vi "LSMcontroller_v64_updatedwaveformhandling.vi"() -> ()   [LabVIEW 2015] (continued)
                        n4774 = call "correctwaveformsizetemp.vi"("new sampling frequency (Hz)"=w1792, "start"=FALSE, "reference waveforms to"=w1800, "Analog waveforms in"=w1807, "stop"=FALSE, "Digital waveforms in"=w1799) -> ("analog wf out"=w1803:waveform(dbl)[], "Digital wf out"=w1801:digitalwaveform[], "measpoints"=w1794:i32)
                        n4775 = local write "Analog Lines Plot"(w1803) -> ()
                        n4776 = call "GetNumCamFramesv2.vi"("Digital Waveform Graph"=w1801) -> ("Numeric"=w1802:i32)  [unwired: 10 in]
                        n4777 = local write "Digital Lines Plot"(w1801) -> ()
                        n4778 = case shown="True" w1795 {
                          tunnel: w1794 -> [_ w1815]
                          frame False {
                          }
                          frame True {
                            n4779 = local write "# of frames"(w1815) -> ()
                          }
                        }
                        n4780 = call "waveformsAObuffer.vi"("AO wf in"=w1803, "command"="set") -> ()  [unwired: 1 out]
                        n4781 = call "waveformsDObuffer.vi"("DO wf in"=w1801, "command"="set") -> ()  [unwired: 1 out]
                        n4782 = local write "Total Camera Frames"(w1802) -> ()
                      }
                    }
                  }
                  frame #4 {
                    w1817 = FALSE ("addAO")
                    n4783 = local read "finite samples"() -> (w1818:bool)
                    n4784 = local read "continuous"() -> (w1819:bool)
                    n4785 = local read "wavdet"() -> (w1820:bool)
                    n4786 = call "2pparameters.vi"("command"="get") -> ("params out"=w1823:T10)  [unwired: 1 in]
                    n4787 = Bundle By Name(cluster=w1823, "finite"=w1818, "cont"=w1819, "wavdet"=w1820) -> (w1821:T10)
                    n4788 = local write "not loadedDOml"(FALSE ("not loadedDO")) -> ()
                    n4789 = local write "changeDOmatlab"(w1817) -> ()
                    n4790 = property on="Load Matlab Waveform DO" class="Bool (strict)"("Val(Sgnl)"=w1817) -> ()  [unwired: 2 in, 2 out]
                    n4791 = call "2pparameters.vi"("Params in"=w1821, "command"="set") -> ()  [unwired: 1 out]
                  }
                }
              }
            }
          }
          event "Add settings": Value Change {
            n4792 = event-data() -> ("NewVal"=w1825:bool)  [unwired: 1 in, 5 out]
            n4793 = case shown="True" w1825 {
              frame False {
              }
              frame True {
                n4794 = stacked-sequence {
                  frame #0 {
                    n4795 = call "wfsettings.vi"("command"="get") -> ("wfsettings out"=w1828:T27)  [unwired: 2 in, 1 out]
                    n4796 = in-place {
                      n4797 = in-place-cluster #53(w1828) -> ("settings names"=w1833:string[], "settings locations"=w1835:path[])
                      n4798 = local read "Setting location"() -> (w1831:path)
                      n4799 = local read "Nickname"() -> (w1830:string)
                      n4800 = Build Array (concatenate)(w1833, w1830) -> (w1832:string[])
                      n4801 = property on="Loaded settings" class="Ring (strict)"("Strings []"=w1832) -> ()  [unwired: 2 in, 2 out]
                      n4802 = Build Array (concatenate)(w1835, w1831) -> (w1834:path[])
                      n4803 = in-place-cluster #53("settings names"=w1832, "settings locations"=w1834) -> (w1826:T27)
                    }
                    n4804 = call "wfsettings.vi"("wfsettings in"=w1826, "command"="set") -> ()  [unwired: 1 in, 2 out]
                  }
                  frame #1 {
                    n4805 = property on="Add settings" class="Bool (strict)"("Val(Sgnl)"=FALSE ("Value (Signaling)")) -> ()  [unwired: 2 in, 2 out]
                  }
                }
              }
            }
          }
          event "Rem setting": Value Change {
            n4806 = event-data() -> ("NewVal"=w1837:bool)  [unwired: 1 in, 5 out]
            n4807 = case shown="True" w1837 {
              frame False {
              }
              frame True {
                n4808 = stacked-sequence {
                  frame #0 {
                    n4809 = call "wfsettings.vi"("command"="get") -> ("wfsettings out"=w1840:T27)  [unwired: 2 in, 1 out]
                    n4810 = in-place {
                      n4811 = in-place-cluster #54(w1840) -> ("settings names"=w1845:string[], "settings locations"=w1843:path[])
                      n4812 = property on="Loaded settings" class="Ring (strict)"() -> ("RingText.Text"=w1846:string)  [unwired: 2 in, 2 out]
                      n4813 = Search 1D Array(1D array=w1845, element=w1846) -> (index of element=w1847:i32)  [unwired: 1 in]
                      n4814 = Delete From Array(array=w1845, index=w1847) -> (array with subset deleted=w1844:string[])  [unwired: 1 in, 1 out]
                      n4815 = Delete From Array(array=w1843, index=w1847) -> (array with subset deleted=w1842:path[])  [unwired: 1 in, 1 out]
                      n4816 = property on="Loaded settings" class="Ring (strict)"("Strings []"=w1844) -> ()  [unwired: 2 in, 2 out]
                      n4817 = in-place-cluster #54("settings names"=w1844, "settings locations"=w1842) -> (w1838:T27)
                    }
                    n4818 = call "wfsettings.vi"("wfsettings in"=w1838, "command"="set") -> ()  [unwired: 1 in, 2 out]
                  }
                  frame #1 {
                    n4819 = property on="Rem setting" class="Bool (strict)"("Val(Sgnl)"=FALSE ("Value (Signaling)")) -> ()  [unwired: 2 in, 2 out]
                  }
                }
              }
            }
          }
          event "Update settings": Value Change {
            n4820 = event-data() -> ("NewVal"=w1849:bool)  [unwired: 1 in, 5 out]
            n4821 = case shown="True" w1849 {
              frame False {
              }
              frame True {
                n4822 = stacked-sequence {
                  frame #0 {
                    n4823 = local read "Measurement"() -> (w1850:T4)
                    n4824 = case shown="\"Timetrace\"" w1850 {
                      frame "X-Y-t movie", Default {
                        n4825 = local read "avpp"() -> (w1871:i32)
                        n4826 = local read "Angle ref"() -> (w1870:dbl)
                        n4827 = local read "ROI Type"() -> (w1869:u16)
                        n4828 = local read "xpixels ref"() -> (w1866:i32)
                        n4829 = local read "Vx-min ref"() -> (w1865:dbl)
                        n4830 = local read "Vx-max ref"() -> (w1864:dbl)
                        n4831 = local read "ypixels ref"() -> (w1862:i32)
                        n4832 = local read "Vy-min ref"() -> (w1863:dbl)
                        n4833 = local read "Vy-max ref"() -> (w1859:dbl)
                        n4834 = local read "Sampling rate"() -> (w1853:dbl)
                        n4835 = local read "finite samples"() -> (w1854:bool)
                        n4836 = local read "continuous"() -> (w1857:bool)
                        n4837 = local read "wavdet"() -> (w1858:bool)
                        n4838 = local read "# of frames"() -> (w1856:i32)
                        n4839 = local read "maxbufferAI"() -> (w1855:i32)
                        n4840 = local read "Override AI buffer"() -> (w1851:bool)
                        n4841 = call "2pparameters.vi"("command"="get") -> ("params out"=w1868:T10)  [unwired: 1 in]
                        n4842 = Bundle By Name(cluster=w1868, "type"="X-Y-t movie", "avpp"=w1871, "Angle Img"=w1870, "Xpixels Img"=w1866, "Vx-min Img"=w1865, "VX-max Img"=w1864, "Ypixels Img"=w1862, "Vy-min Img"=w1863, "Vy-max Img"=w1859, "srate"=w1853, "srate Img"=w1853, "finite"=w1854, "cont"=w1857, "wavdet"=w1858, "measpoints"=w1856, "maxbufferAI"=w1855, "Drawing Mode"=w1869, "Vz-reset"=0.0, "AIoverride"=w1851) -> (w1860:T10)
                        n4843 = call "2pparameters.vi"("Params in"=w1860, "command"="set") -> ()  [unwired: 1 out]
                      }
                      frame "X-Y-Z stack" {
                        n4844 = call "2pparameters.vi"("command"="get") -> ("params out"=w1875:T10)  [unwired: 1 in]
                        n4845 = Bundle By Name(cluster=w1875, "type"="X-Y-Z stack") -> (w1873:T10)
                        n4846 = call "2pparameters.vi"("Params in"=w1873, "command"="set") -> ()  [unwired: 1 out]
                      }
                      frame "Lifetime (scan)" {
                        n4847 = call "2pparameters.vi"("command"="get") -> ("params out"=w1880:T10)  [unwired: 1 in]
                        n4848 = Bundle By Name(cluster=w1880, "type"="Lifetime (scan)") -> (w1878:T10)
                        n4849 = call "2pparameters.vi"("Params in"=w1878, "command"="set") -> ()  [unwired: 1 out]
                      }
                      frame "Lifetime (contour)" {
                        n4850 = local read "Vy-min draw"() -> (w1890:dbl)
                        n4851 = local read "Vy-max draw"() -> (w1889:dbl)
                        n4852 = local read "Vx-min draw"() -> (w1892:dbl)
                        n4853 = local read "Vx-max draw"() -> (w1891:dbl)
                        n4854 = local read "xpixels ref"() -> (w1888:i32)
                        n4855 = local read "ypixels ref"() -> (w1887:i32)
                        n4856 = local read "ROI Type"() -> (w1886:u16)
                        n4857 = local read "srateAODOtt"() -> (w1897:dbl)
                        n4858 = local read "# of frames"() -> (w1902:i32)
                        n4859 = local read "refreshtime"() -> (w1894:dbl)
                        n4860 = local read "Pel"() -> (w1885:dbl)
                        n4861 = local read "bin"() -> (w1900:dbl)
                        n4862 = local read "Override AI buffer"() -> (w1883:bool)
                        n4863 = local read "finite samples"() -> (w1909:bool)
                        n4864 = local read "srateAODOtt"() -> (w1896:dbl)
                        n4865 = local read "srateAODOtt"() -> (w1903:dbl)
                        n4866 = local read "continuous"() -> (w1908:bool)
                        n4867 = local read "Angle ref"() -> (w1893:dbl)
                        n4868 = local read "wavdet"() -> (w1910:bool)
                        n4869 = local read "Vx-ref"() -> (w1905:dbl)
                        n4870 = local read "Vy-ref"() -> (w1907:dbl)
                        n4871 = local read "avpp"() -> (w1906:i32)
                        n4872 = call "tt_timeandsamples.vi"("bin"=w1900, "refreshtime"=w1894, "srateAODOtt"=w1897, "tot#ofsamples"=w1902) -> ("refreshrate"=w1898:dbl, "refreshbuffer"=w1899:i32, "timetracecycles"=w1904:i32)  [unwired: 5 in]
                        n4873 = local read "bin"() -> (w1901:dbl)
                        n4874 = call "2pparameters.vi"("command"="get") -> ("params out"=w1913:T10)  [unwired: 1 in]
                        n4875 = Bundle By Name(cluster=w1913, "Drawing Mode"=w1886, "measpoints"=w1902, "tt_cycles"=w1904, "refreshbuffer"=w1899, "refreshrate"=w1898, "Vx-ref"=w1905, "Vy-ref"=w1907, "srate"=w1896, "finite"=w1909, "cont"=w1908, "wavdet"=w1910, "avpp"=w1906, "srateAODO"=w1903, "bufferAI"=w1899, "bin"=w1901, "Angle Img"=w1893, "Vxminref"=w1892, "Vxmaxref"=w1891, "Vyminref"=w1890, "Vymaxref"=w1889, "Xpixels Img"=w1888, "Ypixels Img"=w1887, "Pel"=w1885, "Vz-reset"=0.0, "AIoverride"=w1883, "type"="Lifetime (contour)") -> (w1911:T10)
                        n4876 = Reciprocal(x=w1898) -> (1/x=w1895:dbl)
                        n4877 = local write "refreshtime"(w1895) -> ()
                        n4878 = call "2pparameters.vi"("Params in"=w1911, "command"="set") -> ()  [unwired: 1 out]
                      }
                      frame "X-Y-Z-t movie" {
                      }
                      frame "linescan" {
                      }
                      frame "Timetrace" {
                        n4879 = local read "Vy-min draw"() -> (w1923:dbl)
                        n4880 = local read "Vy-max draw"() -> (w1922:dbl)
                        n4881 = local read "Vx-min draw"() -> (w1925:dbl)
                        n4882 = local read "Vx-max draw"() -> (w1924:dbl)
                        n4883 = local read "xpixels ref"() -> (w1921:i32)
                        n4884 = local read "ypixels ref"() -> (w1920:i32)
                        n4885 = local read "ROI Type"() -> (w1919:u16)
                        n4886 = local read "srateAODOtt"() -> (w1930:dbl)
                        n4887 = local read "# of frames"() -> (w1935:i32)
                        n4888 = local read "refreshtime"() -> (w1927:dbl)
                        n4889 = local read "Pel"() -> (w1918:dbl)
                        n4890 = local read "bin"() -> (w1933:dbl)
                        n4891 = local read "Override AI buffer"() -> (w1916:bool)
                        n4892 = local read "finite samples"() -> (w1942:bool)
                        n4893 = local read "srateAODOtt"() -> (w1929:dbl)
                        n4894 = local read "srateAODOtt"() -> (w1936:dbl)
                        n4895 = local read "continuous"() -> (w1941:bool)
                        n4896 = local read "Angle ref"() -> (w1926:dbl)
                        n4897 = local read "wavdet"() -> (w1943:bool)
                        n4898 = local read "Vx-ref"() -> (w1938:dbl)
                        n4899 = local read "Vy-ref"() -> (w1940:dbl)
                        n4900 = local read "avpp"() -> (w1939:i32)
                        n4901 = call "tt_timeandsamples.vi"("bin"=w1933, "refreshtime"=w1927, "srateAODOtt"=w1930, "tot#ofsamples"=w1935) -> ("refreshrate"=w1931:dbl, "refreshbuffer"=w1932:i32, "timetracecycles"=w1937:i32)  [unwired: 5 in]
                        n4902 = local read "bin"() -> (w1934:dbl)
                        n4903 = call "2pparameters.vi"("command"="get") -> ("params out"=w1946:T10)  [unwired: 1 in]
                        n4904 = Bundle By Name(cluster=w1946, "Drawing Mode"=w1919, "measpoints"=w1935, "tt_cycles"=w1937, "refreshbuffer"=w1932, "refreshrate"=w1931, "Vx-ref"=w1938, "Vy-ref"=w1940, "srate"=w1929, "finite"=w1942, "cont"=w1941, "wavdet"=w1943, "avpp"=w1939, "srateAODO"=w1936, "bufferAI"=w1932, "bin"=w1934, "Angle Img"=w1926, "Vxminref"=w1925, "Vxmaxref"=w1924, "Vyminref"=w1923, "Vymaxref"=w1922, "Xpixels Img"=w1921, "Ypixels Img"=w1920, "Pel"=w1918, "Vz-reset"=0.0, "AIoverride"=w1916, "type"="Timetrace") -> (w1944:T10)
                        n4905 = Reciprocal(x=w1931) -> (1/x=w1928:dbl)
                        n4906 = local write "refreshtime"(w1928) -> ()
                        n4907 = call "2pparameters.vi"("Params in"=w1944, "command"="set") -> ()  [unwired: 1 out]
                      }
                      frame "Lifetime (point)" {
                      }
                    }
                  }
                  frame #1 {
                    w1949 = FALSE ("wavdet")
                    n4908 = call "2pparameters.vi"("command"="get") -> ("params out"=w1953:T10)  [unwired: 1 in]
                    n4909 = Bundle By Name(cluster=w1953, "finite"=w1949, "cont"=w1949, "wavdet"=TRUE) -> (w1950:T10)
                    n4910 = call "2pparameters.vi"("Params in"=w1950, "command"="set") -> ()  [unwired: 1 out]
                  }
                  frame #2 {
                    n4911 = property on="Loaded settings" class="Ring (strict)"() -> ("RingText.Text"=w1955:string)  [unwired: 2 in, 2 out]
                    n4912 = control-ref of="Analog Lines Plot"() -> (w1957:refnum<vi>)
                    n4913 = control-ref of="Digital Lines Plot"() -> (w1956:refnum<vi>)
                    n4914 = call "Usedlinesfromsettingsfile.vi"("sertting"=w1955) -> ("used AO names"=w1961:string[], "used AO lines"=w1960:tag[], "used DO names"=w1959:string[], "used DO lines"=w1958:tag[])
                    n4915 = call "loadAODOwfparamsfromsettingsfile.vi"("sertting"=w1955) -> ()
                    n4916 = call "prepAOWaveplot.vi"("WaveformGraph in"=w1957, "Analog Used Names"=w1961) -> ()  [unwired: 1 in]
                    n4917 = local write "Analog Used Names"(w1961) -> ()
                    n4918 = local write "Analog Used Lines"(w1960) -> ()
                    n4919 = call "prepDOWaveplot.vi"("DigitalGraph in"=w1956, "used DO names"=w1959) -> ()  [unwired: 1 in]
                    n4920 = local write "Digital Used Names"(w1959) -> ()
                    n4921 = local write "Digital Used Lines"(w1958) -> ()
                  }
                  frame #3 {
                    n4922 = call "waveformparamsv2.vi"("command"="get") -> ("Params out"=w1978:T14)  [unwired: 4 in, 2 out]
                    n4923 = Unbundle By Name(w1978) -> ("AO parameters"=w1979:T15, "DO parameters"=w1980:T17)
                    n4924 = for {
                      tunnel: w1979 -> [w2000] mode=indexing
                      tunnel: [w1998] -> w1981 mode=indexing
                      tunnel: [w1997] -> w1966 mode=indexing
                      tunnel: [w1995] -> w1969 mode=indexing
                      i -> [w1999]
                      n4925 = Unbundle By Name(w2000) -> ("AOtab"=w2001:dbl)
                      n4926 = To Long Integer(number=w2001) -> (32bit integer=w1994:i32)
                      n4927 = case shown="2" w1994 {
                        tunnel: w2000 -> [_ w2012 w2014 w2016]
                        tunnel: [_ w2011 w2013 w2015] -> w1996
                        frame -1 {
                        }
                        frame 0, Default {
                          n4928 = call "generateRampedSquareWave_fromAOparameters.vi"("AO params"=w2012) -> ("Waveform"=w2011:waveform(dbl))  [unwired: 1 out]
                        }
                        frame 1 {
                          n4929 = call "generateTriWave_fromAOparameters.vi"("AO params"=w2014) -> ("Waveform"=w2013:waveform(dbl))  [unwired: 1 out]
                        }
                        frame 2 {
                          n4930 = call "matlabAOwffromparam.vi"("Cluster"=w2016) -> ("Waveform"=w2015:waveform(dbl))  [unwired: 1 out]
                        }
                      }
                      n4931 = case shown="0" w1999 {
                        tunnel: [w2006 -1] -> w1998
                        tunnel: [w2005 w2009] -> w1997
                        tunnel: w1996 -> [w2005 w2009]
                        tunnel: [w2002 -1.0] -> w1995
                        frame 0 {
                          n4932 = Unbundle By Name(w2005) -> ("dt"=w2004:dbl, "Y"=w2007:dbl[])
                          n4933 = Reciprocal(x=w2004) -> (1/x=w2003:dbl)
                          n4934 = Array Size(array=w2007) -> (size(s)=w2006:i32)
                          n4935 = Round To Nearest(number=w2003) -> (nearest integer value=w2002:dbl)
                        }
                        frame 1, Default {
                        }
                      }
                    }
                    n4936 = Index Array(array=w1981, index=0) -> (element=w1983:i32)
                    n4937 = Index Array(array=w1969, index=0) -> (element=w1968:dbl)
                    n4938 = for {
                      tunnel: w1980 -> [w1988] mode=indexing
                      tunnel: [w1986] -> w1967 mode=indexing
                      tunnel: w1983 -> [w1985]
                      n4939 = Unbundle By Name(w1988) -> ("DOtab"=w1987:dbl)
                      n4940 = case shown="0, Default" w1987 {
                        tunnel: w1988 -> [w1991 w1993]
                        tunnel: w1985 -> [w1990 _]
                        tunnel: [w1989 w1992] -> w1986
                        frame 0, Default {
                          n4941 = call "simple digital from wf params.vi"("waveform params"=w1991, "number of samples"=w1990) -> ("digital waveform"=w1989:digitalwaveform)
                        }
                        frame 1 {
                          n4942 = call "matlabDOwffromparam.vi"("waveform params"=w1993) -> ("digital waveform"=w1992:digitalwaveform)
                        }
                      }
                    }
                    n4943 = property on="refwf" class="Ring (strict)"() -> ("RingText.Text"=w1971:string)  [unwired: 2 in, 2 out]
                    n4944 = call "correctwaveformsizetemp.vi"("new sampling frequency (Hz)"=w1968, "start"=FALSE, "reference waveforms to"=w1971, "Analog waveforms in"=w1966, "stop"=FALSE, "Digital waveforms in"=w1967) -> ("analog wf out"=w1965:waveform(dbl)[], "Digital wf out"=w1964:digitalwaveform[], "measpoints"=w1962:i32)
                    n4945 = local read "wavdet"() -> (w1963:bool)
                    n4946 = case shown="True" w1963 {
                      tunnel: w1962 -> [_ w1984]
                      frame False {
                      }
                      frame True {
                        n4947 = local write "# of frames"(w1984) -> ()
                      }
                    }
                    n4948 = local write "Analog Lines Plot"(w1965) -> ()
                    n4949 = local write "Digital Lines Plot"(w1964) -> ()
                    n4950 = call "GetNumCamFramesv2.vi"("Digital Waveform Graph"=w1964) -> ("Numeric"=w1976:i32)  [unwired: 10 in]
                    n4951 = call "waveformsAObuffer.vi"("AO wf in"=w1965, "command"="set") -> ()  [unwired: 1 out]
                    n4952 = call "waveformsDObuffer.vi"("DO wf in"=w1964, "command"="set") -> ()  [unwired: 1 out]
                    n4953 = local write "Total Camera Frames"(w1976) -> ()
                  }
                  frame #4 {
                    n4954 = local read "AO channels"() -> (w2017:u32)
                    n4955 = call "2pparameters.vi"("command"="get") -> ("params out"=w2019:T10)  [unwired: 1 in]
                    n4956 = Unbundle By Name(w2019) -> ("aAO"=w2018:u32[])
                    n4957 = Search 1D Array(1D array=w2018, element=w2017) -> (index of element=w2021:i32)  [unwired: 1 in]
                    n4958 = Equal?(x=w2021, y=-1.0) -> (x = y?=w2022:bool)
                    n4959 = case shown="False" w2022 {
                      tunnel: w2021 -> [w2047 _]
                      frame False {
                        n4960 = call "waveformparamsv2.vi"("command"="get") -> ("Params out"=w2030:T14)  [unwired: 4 in, 2 out]
                        n4961 = Unbundle By Name(w2030) -> ("AO parameters"=w2029:T15)
                        n4962 = Index Array(array=w2029, index=w2047) -> (element=w2046:T16)
                        n4963 = Unbundle By Name(w2046) -> ("AOtab"=w2027:dbl, "Repeats"=w2045:dbl, "Cycles"=w2044:dbl, "Start amplitude (V)"=w2043:dbl, "Baseline (V)"=w2042:dbl, "Step size (V)"=w2041:dbl, "DC (%)"=w2040:dbl, "Sampling frequency (Hz)"=w2039:dbl, "Period (ms)"=w2038:dbl, "Offset (V)"=w2037:dbl, "Amplitude (V)"=w2036:dbl, "Frequency"=w2035:dbl, "Tri Repeats"=w2034:dbl, "phase shift (ms)"=w2033:dbl, "Pulses"=w2032:dbl, "Tri phase"=w2028:dbl, "padding value"=w2024:dbl, "Matlab wave file"=w2025:path)
                        n4964 = To Unsigned Long Integer(number=w2027) -> (unsigned 32bit integer=w2026:u32)
                        n4965 = local write "Build analog waveform tabs"(w2026) -> ()
                        n4966 = local write "Matlab waveform path"(w2025) -> ()
                        n4967 = local write "phase shift (ms)"(w2033) -> ()
                        n4968 = local write "Repeats"(w2045) -> ()
                        n4969 = local write "Cycles"(w2044) -> ()
                        n4970 = local write "Amplitude (V)"(w2036) -> ()
                        n4971 = local write "Matlab padding value"(w2024) -> ()
                        n4972 = local write "Tri padding value"(w2024) -> ()
                        n4973 = local write "Start amplitude (V)"(w2043) -> ()
                        n4974 = local write "Tri Phase (s)"(w2028) -> ()
                        n4975 = local write "Period (ms)"(w2038) -> ()
                        n4976 = local write "Tri Repeats"(w2034) -> ()
                        n4977 = local write "Offset (V)"(w2037) -> ()
                        n4978 = local write "Frequency"(w2035) -> ()
                        n4979 = local write "Pulses"(w2032) -> ()
                        n4980 = local write "padding value"(w2024) -> ()
                        n4981 = local write "Sampling rate \ncurrent wf"(w2039) -> ()
                        n4982 = local write "Baseline (V)"(w2042) -> ()
                        n4983 = local write "Step size (V)"(w2041) -> ()
                        n4984 = local write "DC (%)"(w2040) -> ()
                      }
                      frame True {
                      }
                    }
                  }
                  frame #5 {
                    n4985 = local read "DO channels"() -> (w2050:u16)
                    n4986 = call "2pparameters.vi"("command"="get") -> ("params out"=w2052:T10)  [unwired: 1 in]
                    n4987 = Unbundle By Name(w2052) -> ("aDO"=w2051:u32[])
                    n4988 = Search 1D Array(1D array=w2051, element=w2050) -> (index of element=w2049:i32)  [unwired: 1 in]
                    n4989 = Equal?(x=w2049, y=-1.0) -> (x = y?=w2048:bool)
                    n4990 = case shown="False" w2048 {
                      tunnel: w2049 -> [w2067 _]
                      frame False {
                        n4991 = call "waveformparamsv2.vi"("command"="get") -> ("Params out"=w2061:T14)  [unwired: 4 in, 2 out]
                        n4992 = Unbundle By Name(w2061) -> ("DO parameters"=w2059:T17)
                        n4993 = Index Array(array=w2059, index=w2067) -> (element=w2066:T18)
                        n4994 = Unbundle By Name(w2066) -> ("Digital DC (%)"=w2065:dbl, "Digital phase"=w2064:dbl, "Digital Freq (Hz)"=w2063:dbl, "Sampling frequency (Hz)"=w2062:dbl, "Digital time offset (s)"=w2058:dbl, "padding value"=w2057:dbl, "matlab wave file"=w2056:path, "DOtab"=w2055:dbl)
                        n4995 = local write "Build digital waveform tabs"(w2055) -> ()
                        n4996 = local write "Digital DC (%)"(w2065) -> ()
                        n4997 = local write "Matlab waveform path DO"(w2056) -> ()
                        n4998 = local write "Sampling rate \ncurrent wf"(w2062) -> ()
                        n4999 = local write "Digital time offset (s)"(w2058) -> ()
                        n5000 = local write "Matlab padding value DO"(w2057) -> ()
                        n5001 = local write "Digital padding value"(w2057) -> ()
                        n5002 = local write "Digital Freq (Hz)"(w2063) -> ()
                        n5003 = local write "Digital phase (s)"(w2064) -> ()
                      }
                      frame True {
                      }
                    }
                  }
                  frame #6 {
                    n5004 = local read "finite samples"() -> (w2069:bool)
                    n5005 = local read "continuous"() -> (w2070:bool)
                    n5006 = local read "wavdet"() -> (w2071:bool)
                    n5007 = call "2pparameters.vi"("command"="get") -> ("params out"=w2074:T10)  [unwired: 1 in]
                    n5008 = Bundle By Name(cluster=w2074, "finite"=w2069, "cont"=w2070, "wavdet"=w2071) -> (w2072:T10)
                    n5009 = property on="Update settings" class="Bool (strict)"("Val(Sgnl)"=FALSE ("Value (Signaling)")) -> ()  [unwired: 2 in, 2 out]
                    n5010 = call "2pparameters.vi"("Params in"=w2072, "command"="set") -> ()  [unwired: 1 out]
                  }
                }
              }
            }
          }
          event "Digital phase (s)", "Digital DC (%)", "Digital Freq (Hz)", "Digital padding value", "Digital time offset (s)": Value Change {
            n5011 = event-data() -> ()  [unwired: 1 in, 6 out]
            n5012 = local write "not loadedDO"(TRUE ("not loadedDO")) -> ()
          }
          event "Matlab padding value DO", "Matlab waveform path DO": Value Change {
            n5013 = event-data() -> ()  [unwired: 1 in, 6 out]
            n5014 = local write "not loadedDOml"(TRUE ("not loadedDO")) -> ()
          }
          event "phase shift (ms)", "Pulses", "Baseline (V)", "Step size (V)", "Start amplitude (V)", "Period (ms)", "DC (%)", "Cycles", "Repeats", "padding value": Value Change {
            n5015 = event-data() -> ()  [unwired: 1 in, 6 out]
            n5016 = local write "not loaded"(TRUE ("not loaded")) -> ()
          }
          event "Tri Repeats", "Amplitude (V)", "Offset (V)", "Frequency", "Tri Phase (s)", "Tri padding value": Value Change {
            n5017 = event-data() -> ()  [unwired: 1 in, 6 out]
            n5018 = local write "not loadedtri"(TRUE ("not loadedtri")) -> ()
          }
          event "Matlab waveform path", "Matlab padding value": Value Change {
            n5019 = event-data() -> ()  [unwired: 1 in, 6 out]
            n5020 = local write "not loadedml"(TRUE ("not loadedml")) -> ()
          }
          event "Exit": Value Change {
            n5021 = event-data() -> ("NewVal"=w2081:bool)  [unwired: 1 in]
          }
        }
        n5022 = Wait (ms)(milliseconds to wait=u32 50) -> ()  [unwired: 1 out]
      }
    }
    frame #3 {
      w6485 = FALSE ("Value (Signaling)")
      n5023 = property on="Start" class="Bool (strict)"("Val(Sgnl)"=w6485) -> ()  [unwired: 2 in, 2 out]
      n5024 = property on="Exit" class="Bool (strict)"("Val(Sgnl)"=w6485) -> ()  [unwired: 2 in, 2 out]
      n5025 = property on="Stop" class="Bool (strict)"("Val(Sgnl)"=w6485) -> ()  [unwired: 2 in, 2 out]
      n5026 = flat-sequence {
        frame #0 {
          w6486 = u16 1 items=["OD 0"=1, "OD 0.5"=2, "OD 1"=3, "OD 2"=4, "OD 3"=5, "OD 4"=6] ("New ODfilt")
          n5027 = local read "ODfilt"() -> (w6487:u16)
          n5028 = call "filterwheelcontrol_nothorlabslib.vi"("Current OD filt"=w6487, "New ODfilt"=w6486) -> ()  [unwired: 1 in]
        }
        frame #1 {
          n5029 = Wait (ms)(milliseconds to wait=u32 1000) -> ()  [unwired: 1 out]
        }
      }
    }
  }
